vi "RuntimeConfigurationManagerExample.vi"() -> ()   [LabVIEW 2026]
uses:
  <vilib>/NI VeriStand/Execution/RuntimeConfiguration/NI_VS RuntimeConfiguration ExecutionAPI.lvlib
panel:
  out "error":errorcluster
  in  "Timeout ms":u32=5000
  in  "stop":bool
  in  "Remove Configuration":bool=TRUE
  in  "Gateway IP Address (\"\": localhost)":string="localhost"
  in  "Apply Configuration":bool=TRUE
  in  "Configuration File Path":path
  in  "Runtime Configurable Section Path":string
  out "error out":errorcluster
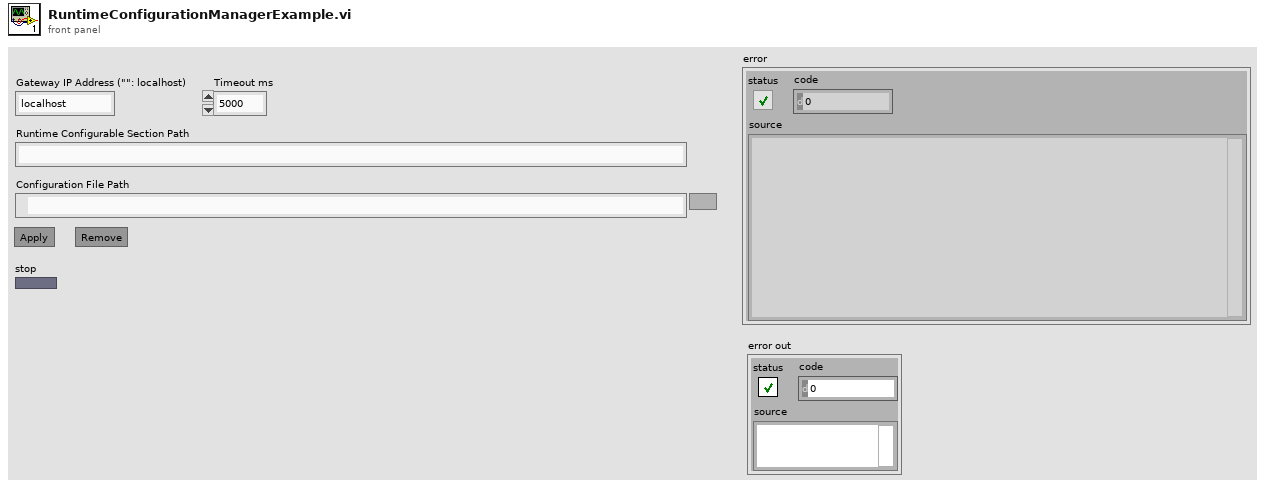
[diagram p1: front panel]
types:
  T1 = typedef "NI_VS RuntimeConfiguration ExecutionAPI.lvlib/Runtime Configuration Manager Ref.ctl" = refnum<k24>
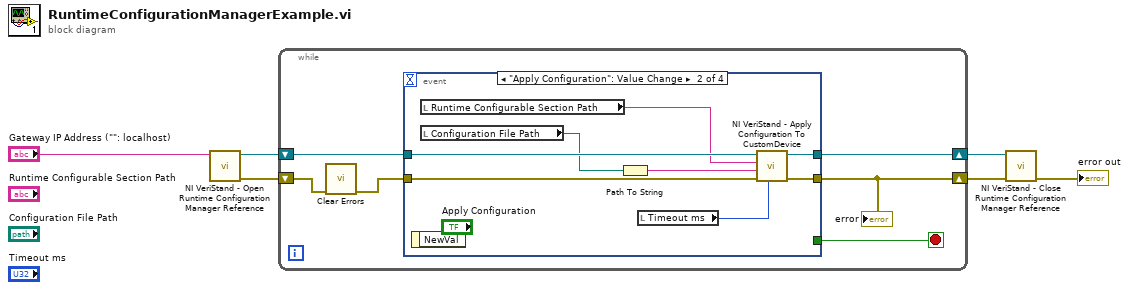
[diagram p0: block diagram]
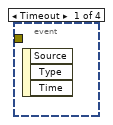
[diagram p2: hidden frame]
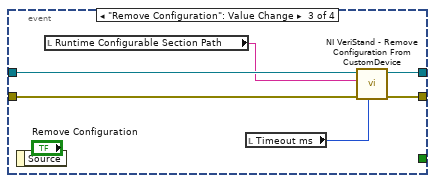
[diagram p3: hidden frame]
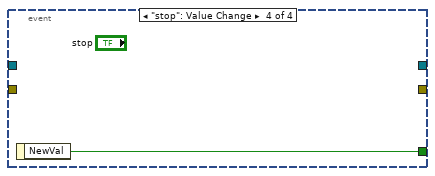
[diagram p4: hidden frame]
diagram:
  n1 = call <vilib>:"NI VeriStand - Open Runtime Configuration Manager Reference.vi"("Gateway IP Address (\"\": localhost)"="Gateway IP Address (\"\": localhost)") -> ("error out"=w5:errorcluster, "Runtime Configuration Manager"=w4:T1)  [unwired: 9 in]
  n2 = while {
    shift-right: [w10] -> w3
    shift-left: w5 -> [w8]
    shift-right: [w11] -> w2
    shift-left: w4 -> [w12]
    stop <- w9 stop-if-true
    n3 = call <vilib>:"Clear Errors.vi"("error in (no error)"=w8) -> ("error out"=w7:errorcluster)  [unwired: 5 in, 1 out]
    n4 = event shown="[1] \"Apply Configuration\": Value Change" {
      selector: _ -> [_ _ _ _]
      dyn-events: _ -> [_ _ _ _]
      timeout: _ -> [_ _ _ _]
      tunnel: w7 -> [_ w20 w24 _]
      tunnel: w12 -> [_ w19 w26 _]
      tunnel: [_ w18 w23 _] -> w10
      tunnel: [_ w17 w25 _] -> w11
      tunnel: [_ _ _ w27] -> w9
      event Timeout {
        n5 = event-data() -> ()  [unwired: 1 in, 3 out]
      }
      event "Apply Configuration": Value Change {
        n6 = event-data() -> ()  [unwired: 1 in, 1 out]
        n7 = local read "Runtime Configurable Section Path"() -> (w16:string)
        n8 = local read "Configuration File Path"() -> (w15:path)
        n9 = Path To String(path=w15) -> (string=w14:string)
        n10 = local read "Timeout ms"() -> (w13:u32)
        n11 = call <vilib>:"NI VeriStand - Apply Configuration To CustomDevice.vi"("Timeout ms"=w13, "error in"=w20, "Configuration File Path"=w14, "Runtime Configurable Section Path"=w16, "Runtime Configuration Manager In"=w19) -> ("error out"=w18:errorcluster, "Runtime Configuration Manager Out"=w17:T1)  [unwired: 5 in]
      }
      event "Remove Configuration": Value Change {
        n12 = event-data() -> ()  [unwired: 1 in, 1 out]
        n13 = local read "Runtime Configurable Section Path"() -> (w21:string)
        n14 = local read "Timeout ms"() -> (w22:u32)
        n15 = call <vilib>:"NI VeriStand - Remove Configuration From CustomDevice.vi"("Timeout ms"=w22, "error in"=w24, "Runtime Configurable Section Path"=w21, "Runtime Configuration Manager In"=w26) -> ("error out"=w23:errorcluster, "Runtime Configuration Manager Out"=w25:T1)  [unwired: 6 in]
      }
      event "stop": Value Change {
        n16 = event-data() -> ("NewVal"=w27:bool)  [unwired: 1 in]
      }
    }
    "error" <- w10
  }
  n17 = call <vilib>:"NI VeriStand - Close Runtime Configuration Manager Reference.vi"("error in"=w3, "Runtime Configuration Manager"=w2) -> ("error out"=→"error out":errorcluster)  [unwired: 9 in]
